vi "SAWLAN_getEVM_Only.vi"(8 "error in":errorcluster, 11 "VISA in":refnum<visa-resource-name>) -> (0 "error out":errorcluster, 1 "All":dbl[](array[numeric]) format="%#.3g", 3 "VISA out":refnum<visa-resource-name>)   [LabVIEW 2023, in "Keysight.lvlib"]
uses:
  Keysight.lvlib
panel:
  out "Response":string
  # "ch"
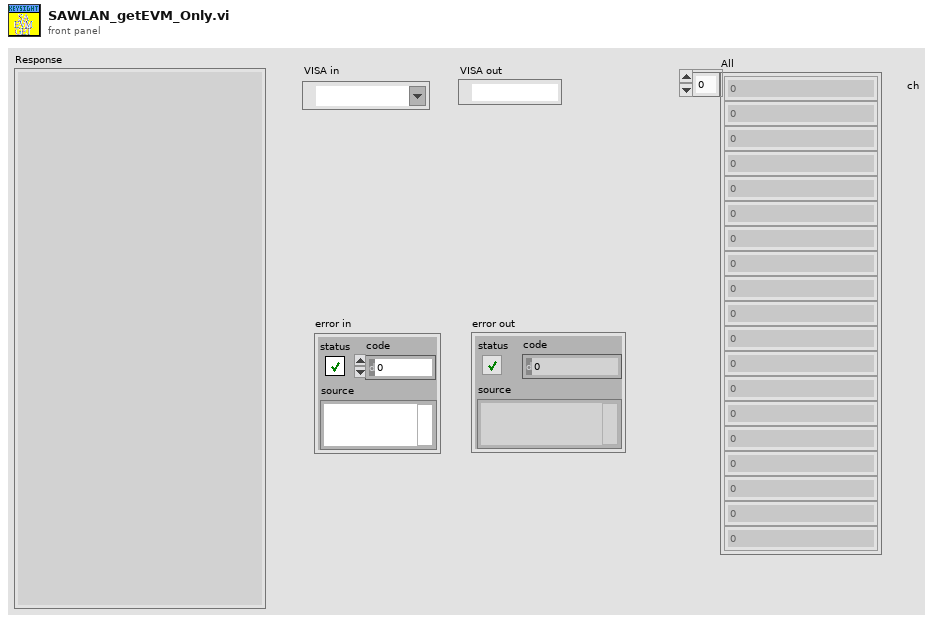
[diagram p1: front panel]
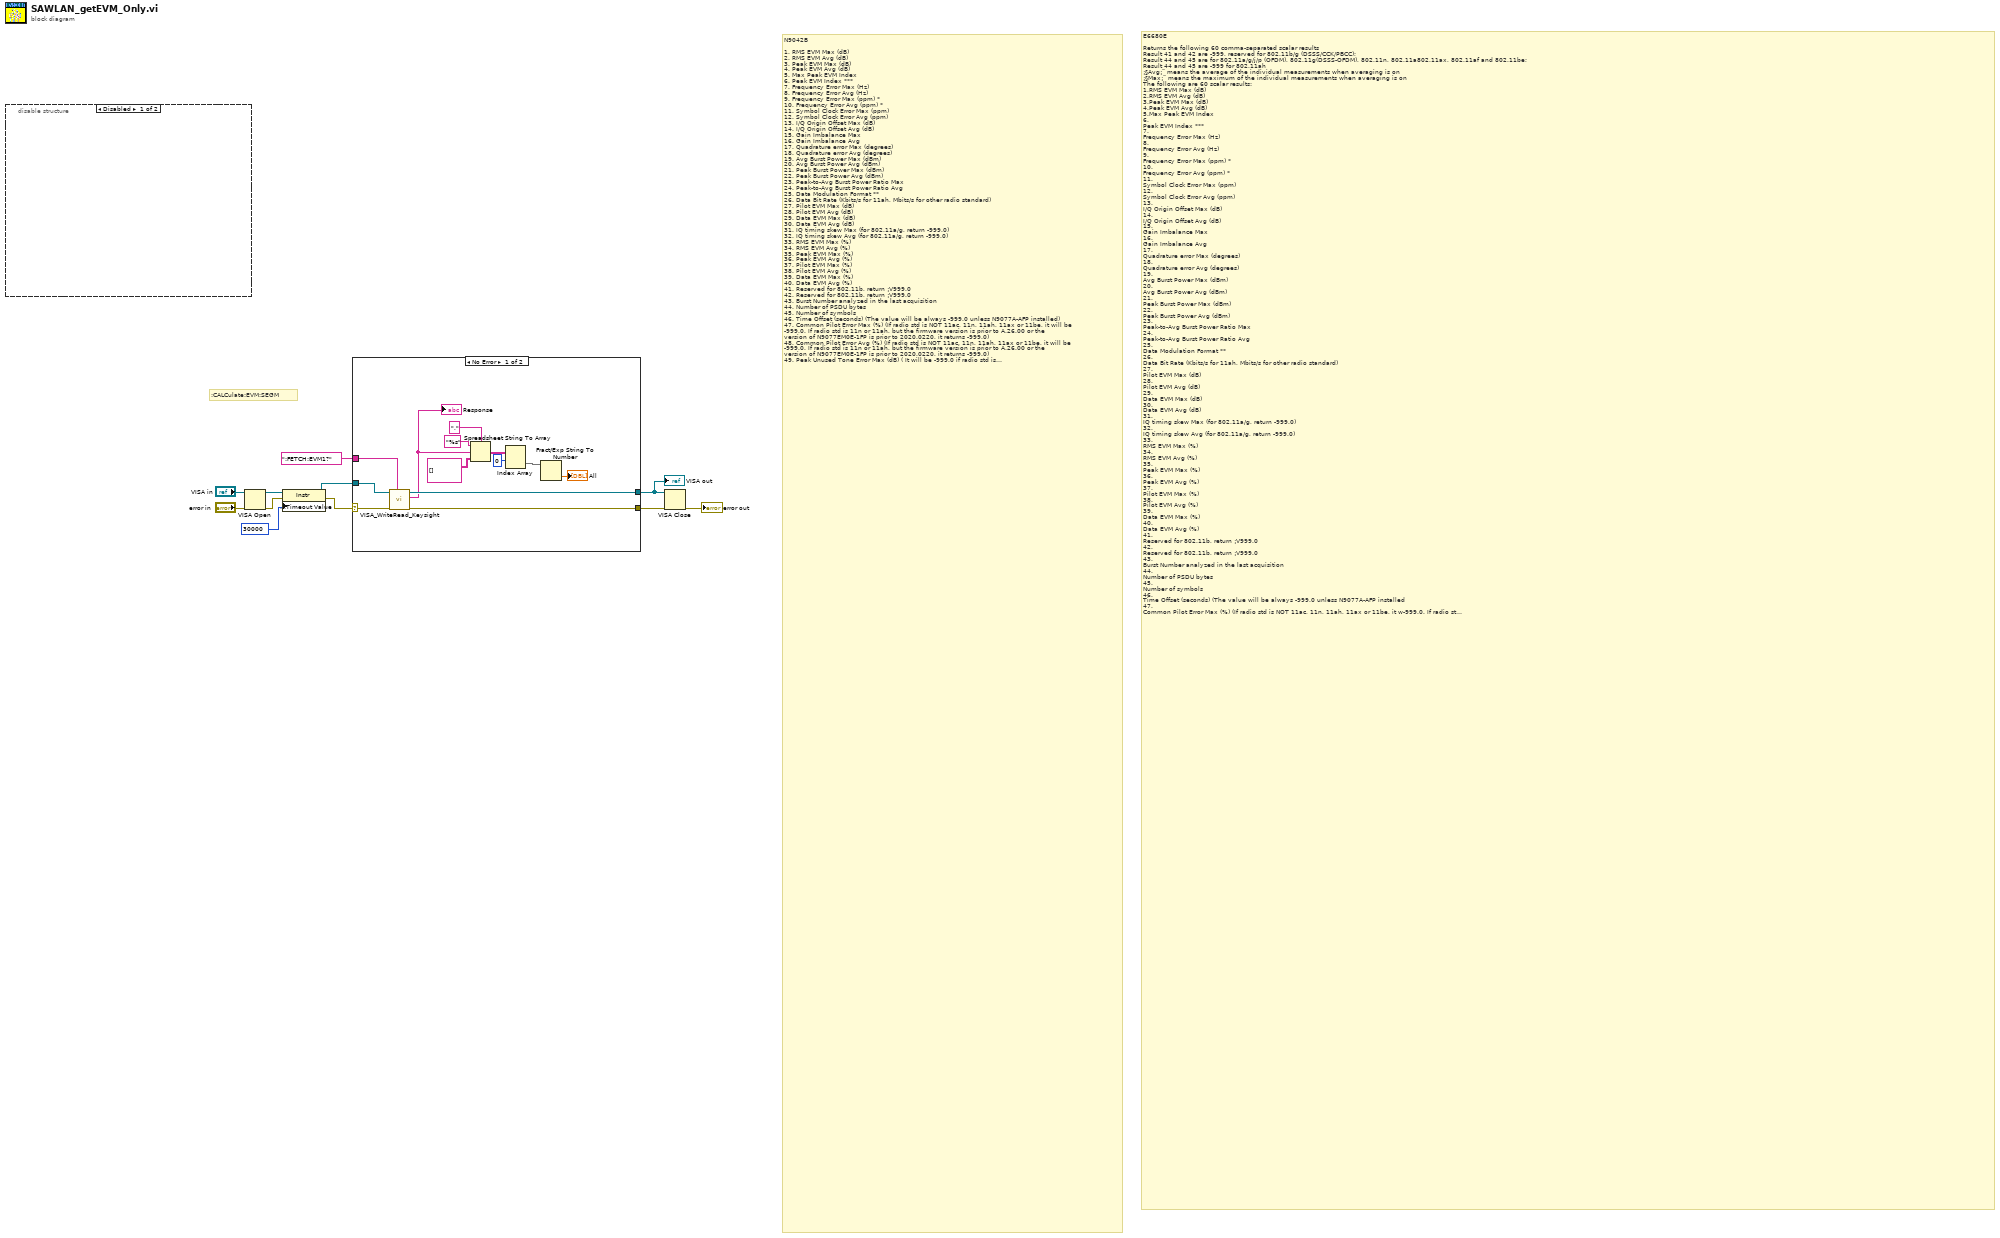
[diagram p0: block diagram]
diagram:
  # ":CALCulate:EVM:SEGM"
  # "E6680E\n\nReturns the following 60 comma-separated scalar results\nResult 41 and 42 are -999, reserved for 802.11b/g (DSSS/CCK/PBCC);\nResult 44 and 45 are for 802.11a/g/j/p (OFDM), 802.11g(DSSS-OFDM), 802.11n, 802.11a802.11ax, 802.11af and 802.11be;\nResult 44 and 45 are -999 for 802.11ah\n¡§Avg¡¨ means the average of the individual measurements when averaging is on\n¡§Max¡¨ means the maximum of the individual measurements when averaging is on\nThe following are 60 scalar results:\n1.RMS EVM Max (dB)\n2.RMS EVM Avg (dB)\n3.Peak EVM Max (dB)\n4.Peak EVM Avg (dB)\n5.Max Peak EVM Index\n6.\nPeak EVM Index ***\n7.\nFrequency Error Max (Hz)\n8.\nFrequency Error Avg (Hz)\n9.\nFrequency Error Max (ppm) *\n10.\nFrequency Error Avg (ppm) *\n11.\nSymbol Clock Error Max (ppm)\n12.\nSymbol Clock Error Avg (ppm)\n13.\nI/Q Origin Offset Max (dB)\n14.\nI/Q Origin Offset Avg (dB)\n15.\nGain Imbalance Max\n16.\nGain Imbalance Avg\n17.\nQuadrature error Max (degrees)\n18.\nQuadrature error Avg (degrees)\n19.\nAvg Burst Power Max (dBm)\n20.\nAvg Burst Power Avg (dBm)\n21.\nPeak Burst Power Max (dBm)\n22.\nPeak Burst Power Avg (dBm)\n23.\nPeak-to-Avg Burst Power Ratio Max\n24.\nPeak-to-Avg Burst Power Ratio Avg\n25.\nData Modulation Format **\n26.\nData Bit Rate (Kbits/s for 11ah, Mbits/s for other radio standard)\n27.\nPilot EVM Max (dB)\n28.\nPilot EVM Avg (dB)\n29.\nData EVM Max (dB)\n30.\nData EVM Avg (dB)\n31.\nIQ timing skew Max (for 802.11a/g, return -999.0)\n32.\nIQ timing skew Avg (for 802.11a/g, return -999.0)\n33.\nRMS EVM Max (%)\n34.\nRMS EVM Avg (%)\n35.\nPeak EVM Max (%)\n36.\nPeak EVM Avg (%)\n37.\nPilot EVM Max (%)\n38.\nPilot EVM Avg (%)\n39.\nData EVM Max (%)\n40.\nData EVM Avg (%)\n41.\nReserved for 802.11b, return ¡V999.0\n42.\nReserved for 802.11b, return ¡V999.0\n43.\nBurst Number analyzed in the last acquisition\n44.\nNumber of PSDU bytes\n45.\nNumber of symbols\n46.\nTime Offset (seconds) (The value will be always -999.0 unless N9077A-AFP installed\n47.\nCommon Pilot Error Max (%) (If radio std is NOT 11ac, 11n, 11ah, 11ax or 11be, it w-999.0. If radio std is 11n or 11ah, but the firmware version is prior to A.26.00 or thversion of N9077EM0E-1FP is prior to 2020.0220, it returns -999.0)\n48.\nCommon Pilot Error Avg (%) (If radio std is NOT 11ac, 11n, 11ah, 11ax or 11be, it w-999.0. If radio std is 11n or 11ah, but the firmware version is prior to A.26.00 or thversion of N9077EM0E-1FP is prior to 2020.0220, it returns -999.0)\n49.\nPeak Unused Tone Error Max (dB) ( It will be -999.0 if radio std is NOT 11ax or 11be\n50.\nPeak Unused Tone Error Avg (dB) ( It will be -999.0 if radio std is NOT 11ax or 11be\n51.\nSymbol Index for Peak Unused Tone Error Max ( It will be -999.0 if radio std is NOT 11be)\n52.\nRu Index for Peak Unused Tone Error Max ( It will be -999.0 if radio std is NOT 11ax11be)\n53.\nHE/EHT PPDU type ( it is 0~6 and will always be -999 if radio std is NOT 11ax or 11b\nFor the 53rd result, HE/EHT PPDU type, the returned integer means:\n0\nHE_SU\n1\nHE_MU\n2\nHE_Extended Range SU\n3\nHE_TriggerBased"
  # "N9042B\n\n1. RMS EVM Max (dB)\n2. RMS EVM Avg (dB)\n3. Peak EVM Max (dB)\n4. Peak EVM Avg (dB)\n5. Max Peak EVM Index\n6. Peak EVM Index ***\n7. Frequency Error Max (Hz)\n8. Frequency Error Avg (Hz)\n9. Frequency Error Max (ppm) *\n10. Frequency Error Avg (ppm) *\n11. Symbol Clock Error Max (ppm)\n12. Symbol Clock Error Avg (ppm)\n13. I/Q Origin Offset Max (dB)\n14. I/Q Origin Offset Avg (dB)\n15. Gain Imbalance Max\n16. Gain Imbalance Avg\n17. Quadrature error Max (degrees)\n18. Quadrature error Avg (degrees)\n19. Avg Burst Power Max (dBm)\n20. Avg Burst Power Avg (dBm)\n21. Peak Burst Power Max (dBm)\n22. Peak Burst Power Avg (dBm)\n23. Peak-to-Avg Burst Power Ratio Max\n24. Peak-to-Avg Burst Power Ratio Avg\n25. Data Modulation Format **\n26. Data Bit Rate (Kbits/s for 11ah, Mbits/s for other radio standard)\n27. Pilot EVM Max (dB)\n28. Pilot EVM Avg (dB)\n29. Data EVM Max (dB)\n30. Data EVM Avg (dB)\n31. IQ timing skew Max (for 802.11a/g, return -999.0)\n32. IQ timing skew Avg (for 802.11a/g, return -999.0)\n33. RMS EVM Max (%)\n34. RMS EVM Avg (%)\n35. Peak EVM Max (%)\n36. Peak EVM Avg (%)\n37. Pilot EVM Max (%)\n38. Pilot EVM Avg (%)\n39. Data EVM Max (%)\n40. Data EVM Avg (%)\n41. Reserved for 802.11b, return ¡V999.0\n42. Reserved for 802.11b, return ¡V999.0\n43. Burst Number analyzed in the last acquisition\n44. Number of PSDU bytes\n45. Number of symbols\n46. Time Offset (seconds) (The value will be always -999.0 unless N9077A-AFP installed)\n47. Common Pilot Error Max (%) (If radio std is NOT 11ac, 11n, 11ah, 11ax or 11be, it will be\n-999.0. If radio std is 11n or 11ah, but the firmware version is prior to A.26.00 or the\nversion of N9077EM0E-1FP is prior to 2020.0220, it returns -999.0)\n48. Common Pilot Error Avg (%) (If radio std is NOT 11ac, 11n, 11ah, 11ax or 11be, it will be\n-999.0. If radio std is 11n or 11ah, but the firmware version is prior to A.26.00 or the\nversion of N9077EM0E-1FP is prior to 2020.0220, it returns -999.0)\n49. Peak Unused Tone Error Max (dB) ( It will be -999.0 if radio std is NOT 11ax or 11be)\n50. Peak Unused Tone Error Avg (dB) ( It will be -999.0 if radio std is NOT 11ax or 11be)\n51. Symbol Index for Peak Unused Tone Error Max ( It will be -999.0 if radio std is NOT 11ax\nor 11be)\n52. Ru Index for Peak Unused Tone Error Max ( It will be -999.0 if radio std is NOT 11ax or\n11be)\n53. HE/EHT PPDU type ( it is 0~6 and will always be -999 if radio std is NOT 11ax or 11be)\nFor the 53rd result, HE/EHT PPDU type, the returned integer means:\n0 HE_SU\n1 HE_MU\n2 HE_Extended Range SU\n3 HE_TriggerBased\n4 HE_SU_Sounding_NDP\n5 HE_TriggerBased_NDP\n6 EHT_MU\n7 EHT_TriggerBased\n8 EHT_Sounding_NDP\n-999 Unknown\n54. Common Pilot Error Max (Degree) (If radio std is NOT 11ac, 11n, 11ah, 11ax or 11be, it\nwill be -999.0. If radio std is 11n or 11ah, but the firmware version is prior to A.26.00 or\nthe version of N9077EM0E-1FP is prior to 2020.0220, it returns -999.0)\n55. Common Pilot Error Avg (Degree) (If radio std is NOT 11ac, 11n, 11ah, 11ax or 11be, it\nwill be -999.0. If radio std is 11n or 11ah, but the firmware version is prior to A.26.00 or\nthe version of N9077EM0E-1FP is prior to 2020.0220, it returns -999.0)\n56. Packet Extension Duration (us) ( it will be -999.0 if radio std is NOT 11ax or 11be)\n57. Guard Interval of Trigger-based PPDU Guard Interval (us) ( it will be -999.0 if radio std is\nNOT 11ax or 11be)\n58. HE-LTF/EHT-LTF type of Trigger-based PPDU if radio std is 11ax/11be; it will be -999.0\nif radio std is NOT 11ax or 11be\nHE-LTF Type of Trigger-based PPDU, the returned integer means:\n0 1 x LTF\n1 2 x LTF\n2 4 x LTF\nEHT-LTF Type of Trigger-based PPDU, the returned integer means:\n1 2 x LTF\n2 4 x LTF\n59. The minimal Meas Interval for successful PSDU CRC decoding (if the Firmware Version\nis below A.22.00, it returns -999.0 which means Invalid)\n60. PSDU CRC for 802.11a/11n/11ac/11af (if the Firmware Version is below A.22.00 or it is\nnot 802.11a/11n/11ac/11af , 1 means Fail, 0 means Pass, -999 means Invalid)\n61. Duty On Period (Unit is microseconds, it is the pulse width, if the Firmware Version is\nbelow A.30.00 or it is not found, it returns -999.0 which means Invalid.-999.0 means\ninvalid)\n62. Duty Off Period (Unit is microseconds, it is (pulse period ¡V pulse width), if the Firmware\nVersion is below A.30.00 or it is not found, it returns -999.0 which means Invalid.)\n63. Duty Cycle (Unit is %, it is pulse width / pulse period, if the Firmware Version is below\nA.30.00 or (either Duty On or Off is not found), it returns -999.0 which means Invalid\n64. Average RMS ccEVM, if the Firmware Version is below A.33.00 or Cross-Correlated\nEVM is off, it returns -999.0 which means Invalid.\nHere ¡§Average¡¨ means using data of each measurement in measurement loop to\ncalculate RMS ccEVM.\nccEVM is not accurate and can¡¦t reflect source EVM if data point is not sufficient, use\nmore data points (average number * Data Points), then it can lead to a more stable and\naccurate ccEVM result.\nIt will not only benefit for the cases that data point is obviously not sufficient (small BW,\nsmall MCS, small symbol length), for all cases, it will lead to a more accurate ccEVM\nresult, the key point is to balance time and improvement\n65. Valid data points that used to calculate ccEVM, if the Firmware Version is below A.33.00\nor ccEVM is off, it returns -999.0 which means Invalid\n66. Total data points that used to calculate ccEVM, if the Firmware Version is below A.33.00\nor ccEVM is off, it returns -999.0 which means Invalid\n67. Partial Burst Power Max (dBm), if the Firmware Version is below A.36 Minor or Radio Std\nis not 11n/ac/ax/be, returns -999.0, which means Invalid. Valid when Radio Std is 11agjp\nif Radio Std Detection is auto, but invalid if Radio Std Detection is Manual\n68. Partial Burst Power Avg(dBm) if the Firmware Version is below A.36 Minor or Radio Std\nis not 11n/ac/ax/be, returns -999.0, which means Invalid. Valid when Radio Std is 11agjp\nif Radio Std Detection is auto, but invalid if Radio Std Detection is Manual"
  n1 = disable-structure shown="Disabled" {
    frame Disabled {
    }
    frame Enabled {
    }
  }
  n2 = VISA Open(error in (no error)="error in", VISA resource name="VISA in") -> (VISA resource name=w4:refnum<visa-resource-name>, error out=w6:errorcluster)  [unwired: 3 in]
  n3 = property on="Property Node" class="Instr"(reference=w4, error in=w6, "General Settings:Timeout Value"=u32 30000) -> (reference out=w8:refnum<visa-resource-name>, error out=w9:errorcluster)
  n4 = case shown="No Error" w9 {
    selector: w9 -> [w20 w26]
    tunnel: [w24 w26] -> w3
    tunnel: [w23 w25] -> w1
    tunnel: ":FETCH:EVM1?" ("write buffer") -> [w22 _]
    tunnel: w8 -> [w21 w25]
    frame No Error {
      n5 = call "VISA_WriteRead_Keysight.vi"("VISA_CMD"=w22, "error in"=w20, "VISA in"=w21) -> ("error out"=w24:errorcluster, "Response"=w14:string, "VISA out"=w23:refnum<visa-resource-name>)  [unwired: 6 in]
      "Response" <- w14
      n6 = Spreadsheet String To Array(delimiter (Tab)="," ("format string"), format string="%s", spreadsheet string=w14, array type (2D Dbl)=string[][] [] ("Array")) -> (array=w19:string[][])
      n7 = Index Array(array=w19, index (row)=0) -> (element=w13:string[])  [unwired: 1 in]
      n8 = Fract/Exp String To Number(string=w13) -> (number=→"All":dbl[])  [unwired: 3 in, 1 out]
    }
    frame Error {
    }
  }
  "VISA out" <- w1
  n9 = VISA Close(VISA resource name=w1, error in (no error)=w3) -> (error out=→"error out":errorcluster)
